vi "ma_SML RT Baseband Zoom FFT (complex input) (No State).vi"(0 "x [V]":cdb[](array[numeric]) format="%.6f", 1 "SML RT Baseband Zoom FFT (complex input) state in":T1={"zoom settings state"={"zoom"=1, "stop band attenuation"=enum."120 dB", "alias protect in final transition"=FALSE, "oversampling ratio"=1.0}, "SML Decimation Filter (complex input) state"={"decimation settings state"={"M"=1, "stop band attenuation"=enum."84 dB", "alias protect in transition band"=TRUE, "oversampling ratio"=1.0}, "counter for garbage samples state"=0, "sml_Parameter Setting for Zoom Factor state"={"filter length * interpolation state"=0, "interpolation state"=0, "comb filter order state"=0, "CFIR par state"={"h"=[], "M"=0, "N"=0}, "LFIR par state"={"h"=[], "M"=0, "N"=0}, "CIC Stages state"=0}, "aal_CIC (complex input) state"={"aal_cascaded moving average (complex input) state"={"states"=[], "circular buffers state"=[], "circular buffer counter state"=0}, "aal_moving average with decimation by order (complex input) state"={"residue result state"=0.0+0.0i, "processed data counter state"=0}}, "sml_Cascaded Decimation Filter (complex input) CFIR state"={"unprocessed data state"=[], "final conditions state"=[], "sml_M-1 Decimator with IC (complex input) state"={"coefficients in reverse order state"=[], "max index for coefficients state"=1}}, "sml_Cascaded Decimation Filter (complex input) LFIR state"={"unprocessed data state"=[], "final conditions state"=[], "sml_M-1 Decimator with IC (complex input) state"={"coefficients in reverse order state"=[], "max index for coefficients state"=1}}}, "ma_SML Data Packing (complex input) state"={"array getting packed state"=[], "last array processed state"=[], "index state"=0, "packing parameters state"={0, "size"=0}}} {"SML Decimation Filter (complex input) state"."sml_Cascaded Decimation Filter (complex input) LFIR state"."sml_M-1 Decimator with IC (complex input) state"."coefficients in reverse order state" format="%.2f"; "SML Decimation Filter (complex input) state"."sml_Cascaded Decimation Filter (complex input) CFIR state"."sml_M-1 Decimator with IC (complex input) state"."coefficients in reverse order state" format="%.2f"; "SML Decimation Filter (complex input) state"."sml_Parameter Setting for Zoom Factor state"."LFIR par state"."h" format="%.2f"; "SML Decimation Filter (complex input) state"."sml_Parameter Setting for Zoom Factor state"."CFIR par state"."h" format="%.2f"; "SML Decimation Filter (complex input) state"."decimation settings state"."oversampling ratio" format="%.2f"; "SML Decimation Filter (complex input) state"."decimation settings state"."M" min=0; "zoom settings state"."oversampling ratio" format="%.2f"; "zoom settings state"."zoom" min=0}, 5 "zoom settings":T3={"zoom"=1, "stop band attenuation"=enum."120 dB", "alias protect in final transition"=FALSE, "oversampling ratio"=1.0} {"oversampling ratio" format="%.2f"; "zoom" min=0}, 7 "FFT settings":T4={"window"=1, "Window Size"=1024, "FFT Size"=1024, "%overlap"=0.0} {"window" items=["Rectangle"=0, "Hanning"=1, "Hamming"=2, "Blackman-Harris"=3, "Exact Blackman"=4, "Blackman"=5, "Flat Top"=6, "4 Term B-Harris "=7, "7 Term B-Harris"=8, "Low Sidelobe"=9, "Blackman Nuttall"=11, "Triangle"=30, "Bartlett-Hanning"=31, "Bohman"=32, "Parzen"=33, "Welch"=34, "Kaiser"=60, "Dolph-Chebyshev"=61, "Gaussian"=62]; "%overlap" min=0.0 max=100.0 format="%.2f"}, 11 "error in (no error)":errorcluster, 12 "reset?":bool) -> (3 "SML RT Baseband Zoom FFT (complex input) state out":T1={"zoom settings state"={"zoom"=1, "stop band attenuation"=enum."120 dB", "alias protect in final transition"=FALSE, "oversampling ratio"=1.0}, "SML Decimation Filter (complex input) state"={"decimation settings state"={"M"=1, "stop band attenuation"=enum."84 dB", "alias protect in transition band"=TRUE, "oversampling ratio"=1.0}, "counter for garbage samples state"=0, "sml_Parameter Setting for Zoom Factor state"={"filter length * interpolation state"=0, "interpolation state"=0, "comb filter order state"=0, "CFIR par state"={"h"=[], "M"=0, "N"=0}, "LFIR par state"={"h"=[], "M"=0, "N"=0}, "CIC Stages state"=0}, "aal_CIC (complex input) state"={"aal_cascaded moving average (complex input) state"={"states"=[], "circular buffers state"=[], "circular buffer counter state"=0}, "aal_moving average with decimation by order (complex input) state"={"residue result state"=0.0+0.0i, "processed data counter state"=0}}, "sml_Cascaded Decimation Filter (complex input) CFIR state"={"unprocessed data state"=[], "final conditions state"=[], "sml_M-1 Decimator with IC (complex input) state"={"coefficients in reverse order state"=[], "max index for coefficients state"=1}}, "sml_Cascaded Decimation Filter (complex input) LFIR state"={"unprocessed data state"=[], "final conditions state"=[], "sml_M-1 Decimator with IC (complex input) state"={"coefficients in reverse order state"=[], "max index for coefficients state"=1}}}, "ma_SML Data Packing (complex input) state"={"array getting packed state"=[], "last array processed state"=[], "index state"=0, "packing parameters state"={0, "size"=0}}} {"SML Decimation Filter (complex input) state"."sml_Cascaded Decimation Filter (complex input) LFIR state"."sml_M-1 Decimator with IC (complex input) state"."coefficients in reverse order state" format="%.2f"; "SML Decimation Filter (complex input) state"."sml_Cascaded Decimation Filter (complex input) CFIR state"."sml_M-1 Decimator with IC (complex input) state"."coefficients in reverse order state" format="%.2f"; "SML Decimation Filter (complex input) state"."sml_Parameter Setting for Zoom Factor state"."LFIR par state"."h" format="%.2f"; "SML Decimation Filter (complex input) state"."sml_Parameter Setting for Zoom Factor state"."CFIR par state"."h" format="%.2f"; "SML Decimation Filter (complex input) state"."decimation settings state"."oversampling ratio" format="%.2f"; "SML Decimation Filter (complex input) state"."decimation settings state"."M" min=0; "zoom settings state"."oversampling ratio" format="%.2f"; "zoom settings state"."zoom" min=0}, 4 "FFT{X} [Vrms]":cdb[](array[numeric]) format="%.6g", 6 "time data":cdb[](array[numeric]) format="%.2f", 8 "spectral info":T2 {"window" items=["Rectangle"=0, "Hanning"=1, "Hamming"=2, "Blackman-Harris"=3, "Exact Blackman"=4, "Blackman"=5, "Flat Top"=6, "4 Term B-Harris "=7, "7 Term B-Harris"=8, "Low Sidelobe"=9, "Blackman Nuttall"=11, "Triangle"=30, "Bartlett-Hanning"=31, "Bohman"=32, "Parzen"=33, "Welch"=34, "Kaiser"=60, "Dolph-Chebyshev"=61, "Gaussian"=62]}, 10 "spectrum ready?":bool, 14 "filter transition length":i32=1 min=0, 15 "error out":errorcluster)   [LabVIEW 2020, in "NI_MAPro.lvlib"]
uses:
  NI_MAPro.lvlib
  ma_sml_Spectral Info.ctl
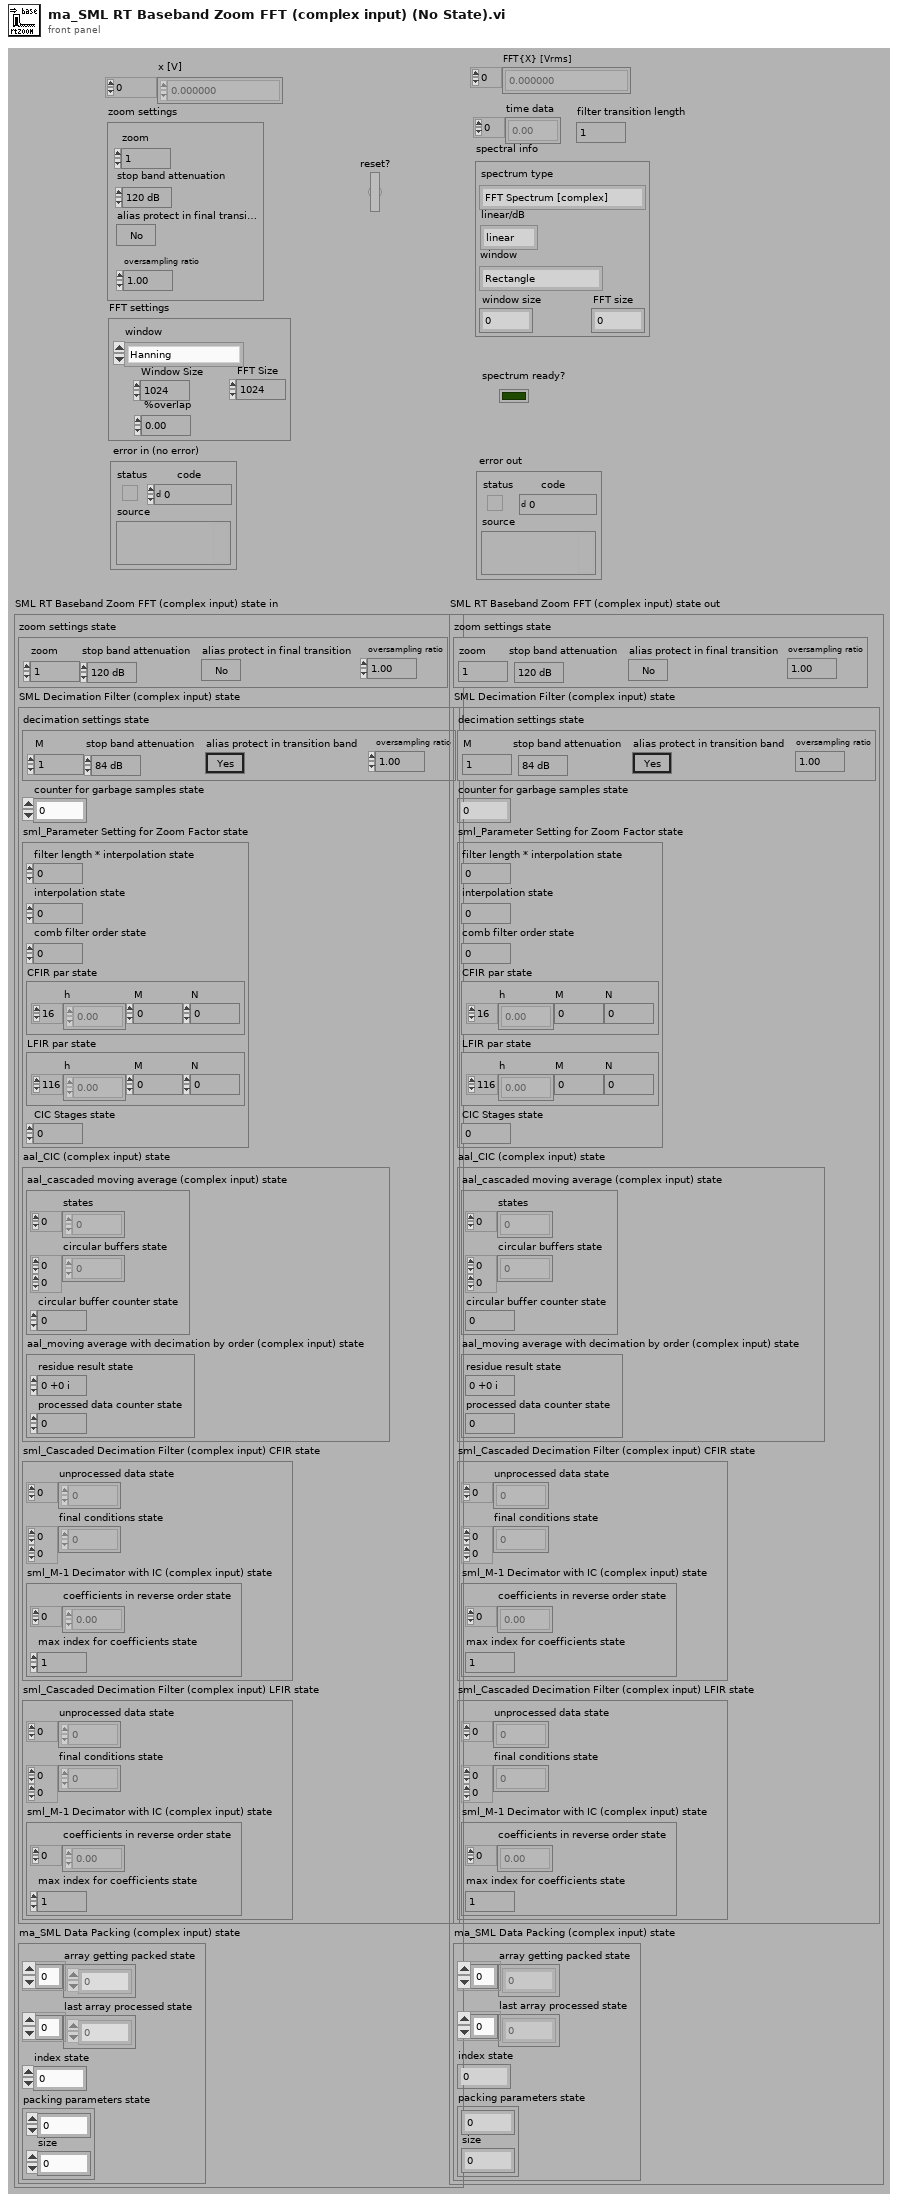
[diagram p1: front panel]
types:
  T1 = cluster{"zoom settings state":cluster{"zoom":i32, "stop band attenuation":enum16{"84 dB", "96 dB", "120 dB"}, "alias protect in final transition":bool, "oversampling ratio":dbl}, "SML Decimation Filter (complex input) state":cluster{"decimation settings state":cluster{"M":i32, "stop band attenuation":enum16{"84 dB", "96 dB", "120 dB"}, "alias protect in transition band":bool, "oversampling ratio":dbl}, "counter for garbage samples state":i32, "sml_Parameter Setting for Zoom Factor state":cluster{"filter length * interpolation state":i32, "interpolation state":i32, "comb filter order state":i32, "CFIR par state":cluster{"h":dbl[], "M":i32, "N":i32}, "LFIR par state":cluster{"h":dbl[], "M":i32, "N":i32}, "CIC Stages state":i32}, "aal_CIC (complex input) state":cluster{"aal_cascaded moving average (complex input) state":cluster{"states":cdb[], "circular buffers state":cdb[][], "circular buffer counter state":i32}, "aal_moving average with decimation by order (complex input) state":cluster{"residue result state":cdb, "processed data counter state":i32}}, "sml_Cascaded Decimation Filter (complex input) CFIR state":cluster{"unprocessed data state":cdb[], "final conditions state":cdb[][], "sml_M-1 Decimator with IC (complex input) state":cluster{"coefficients in reverse order state":dbl[], "max index for coefficients state":i32}}, "sml_Cascaded Decimation Filter (complex input) LFIR state":cluster{"unprocessed data state":cdb[], "final conditions state":cdb[][], "sml_M-1 Decimator with IC (complex input) state":cluster{"coefficients in reverse order state":dbl[], "max index for coefficients state":i32}}}, "ma_SML Data Packing (complex input) state":cluster{"array getting packed state":cdb[], "last array processed state":cdb[], "index state":i32, "packing parameters state":cluster{i32, "size":i32}}}
  T2 = typedef "NI_MAPro.lvlib/ma_sml_Spectral Info.ctl" = cluster{"spectrum type":enum16{"FFT Spectrum [complex]", "Amplitude [Magnitude]", "Power [Magnitude^2]", "Cross Spectrum [complex]", "Frequency Response [Complex]"}, "linear/dB":enum16{"linear", "dB"}, "window":u16, "window size":i32, "FFT size":i32}
  T3 = cluster{"zoom":i32, "stop band attenuation":enum16{"84 dB", "96 dB", "120 dB"}, "alias protect in final transition":bool, "oversampling ratio":dbl}
  T4 = cluster{"window":u16, "Window Size":i32, "FFT Size":i32, "%overlap":dbl}
  T5 = cluster{"array getting packed state":cdb[], "last array processed state":cdb[], "index state":i32, "packing parameters state":cluster{i32, "size":i32}}
  T6 = cluster{"decimation settings state":cluster{"M":i32, "stop band attenuation":enum16{"84 dB", "96 dB", "120 dB"}, "alias protect in transition band":bool, "oversampling ratio":dbl}, "counter for garbage samples state":i32, "sml_Parameter Setting for Zoom Factor state":cluster{"filter length * interpolation state":i32, "interpolation state":i32, "comb filter order state":i32, "CFIR par state":cluster{"h":dbl[], "M":i32, "N":i32}, "LFIR par state":cluster{"h":dbl[], "M":i32, "N":i32}, "CIC Stages state":i32}, "aal_CIC (complex input) state":cluster{"aal_cascaded moving average (complex input) state":cluster{"states":cdb[], "circular buffers state":cdb[][], "circular buffer counter state":i32}, "aal_moving average with decimation by order (complex input) state":cluster{"residue result state":cdb, "processed data counter state":i32}}, "sml_Cascaded Decimation Filter (complex input) CFIR state":cluster{"unprocessed data state":cdb[], "final conditions state":cdb[][], "sml_M-1 Decimator with IC (complex input) state":cluster{"coefficients in reverse order state":dbl[], "max index for coefficients state":i32}}, "sml_Cascaded Decimation Filter (complex input) LFIR state":cluster{"unprocessed data state":cdb[], "final conditions state":cdb[][], "sml_M-1 Decimator with IC (complex input) state":cluster{"coefficients in reverse order state":dbl[], "max index for coefficients state":i32}}}
  T7 = cluster{"zoom":bool, "stop band attenuation":bool, "alias protect in final transition":bool, "oversampling ratio":bool}
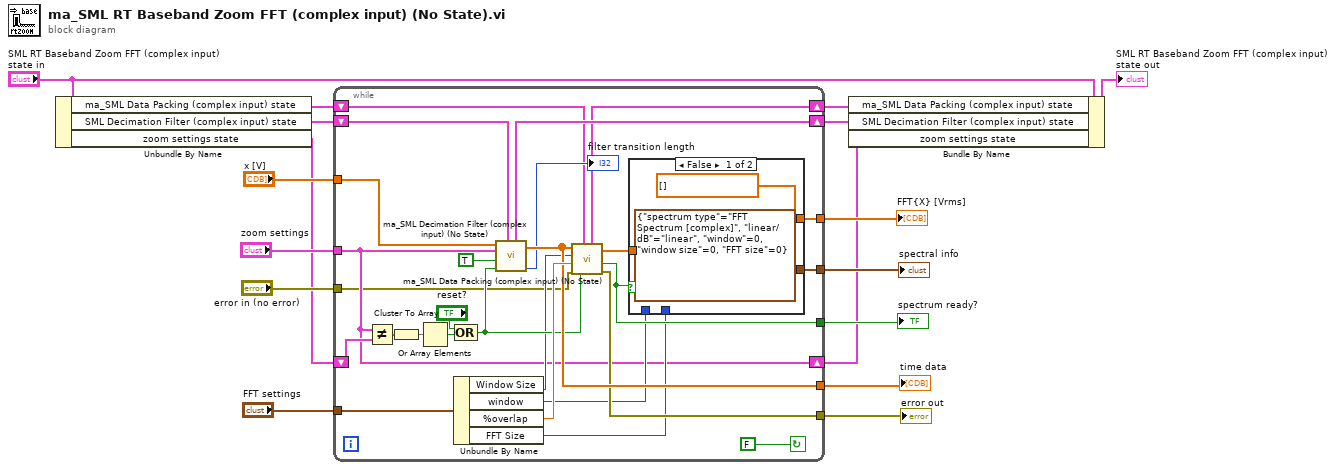
[diagram p0: block diagram]
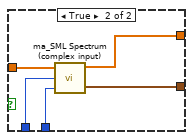
[diagram p2: hidden frame]
diagram:
  n1 = Unbundle By Name("SML RT Baseband Zoom FFT (complex input) state in") -> ("ma_SML Data Packing (complex input) state"=w2:T5, "SML Decimation Filter (complex input) state"=w4:T6, "zoom settings state"=w8:T3)
  n2 = while {
    tunnel: "FFT settings" -> [w22]
    tunnel: "error in (no error)" -> [w23]
    tunnel: [w24] -> w11
    tunnel: "x [V]" -> [w25]
    tunnel: "zoom settings" -> [w26]
    tunnel: [w34] -> w14
    tunnel: [w35] -> w15
    tunnel: [w36] -> w16
    shift-left: w8 -> [w37]
    shift-right: [w26] -> w5
    tunnel: [w44] -> w17
    shift-right: [w20] -> w3
    shift-left: w4 -> [w21]
    shift-right: [w18] -> w1
    shift-left: w2 -> [w19]
    stop <- FALSE continue-if-true
    n3 = Not Equal?(x=w26, y=w37) -> (x != y?=w40:T7)
    n4 = Cluster To Array(cluster=w40) -> (array=w39:bool[])
    n5 = Or Array Elements(Boolean array=w39) -> (logical OR=w42:bool)
    n6 = Unbundle By Name(w22) -> ("Window Size"=w31:i32, "window"=w30:u16, "%overlap"=w41:dbl, "FFT Size"=w29:i32)
    n7 = Compound Arithmetic op=OR("reset?", w42) -> (w33:bool)
    n8 = call "ma_SML Decimation Filter (complex input) (No State).vi"("SML Decimation Filter (complex input) state"=w21, "reset?"=w33, "truncate transition?"=TRUE ("Truncate initial filter Transition"), "decimation setting"=w26, "x"=w25) -> ("initial cutoff length"=→"filter transition length":i32, "y"=w36:cdb[], "SML Decimation Filter (complex input) state"=w20:T6)  [unwired: 4 out]
    n9 = call "ma_SML Data Packing (complex input) (No State).vi"("reset?"=w33, "ma_SML Data Packing (complex input) state"=w19, "error in (no error)"=w23, "%overlap"=w41, "size"=w31, "x"=w36) -> ("error out"=w35:errorcluster, "data ready?"=w44:bool, "y"=w43:cdb[], "ma_SML Data Packing (complex input) state"=w18:T5)  [unwired: 2 out]
    n10 = case shown="False" w44 {
      tunnel: [cdb[] [] ("FFT{x} [Vrms]") w51] -> w34
      tunnel: w43 -> [_ w49]
      tunnel: w30 -> [_ w50]
      tunnel: w29 -> [_ w48]
      tunnel: [T2 {"spectrum type"=enum."FFT Spectrum [complex]", "linear/dB"=enum."linear", "window"=0, "window size"=0, "FFT size"=0} ("spectral info") w47] -> w24
      frame False {
      }
      frame True {
        n11 = call "ma_SML Spectrum (complex input).vi"("FFT size"=w48, "window"=w50, "x [V]"=w49) -> ("spectral info"=w47:T2, "FFT{x} [Vrms]"=w51:cdb[])
      }
    }
  }
  "spectrum ready?" <- w17
  "FFT{X} [Vrms]" <- w14
  "time data" <- w16
  "error out" <- w15
  "spectral info" <- w11
  n12 = Bundle By Name(cluster="SML RT Baseband Zoom FFT (complex input) state in", "ma_SML Data Packing (complex input) state"=w1, "SML Decimation Filter (complex input) state"=w3, "zoom settings state"=w5) -> (→"SML RT Baseband Zoom FFT (complex input) state out":T1)
